vi "LV SCISDK Read Digitizer Data.vi"(8 "error in (no error)":errorcluster, 9 "handle":u64, 11 "Path":string) -> (0 "error out":errorcluster, 1 "handle out":u64, 2 "buffer out":T1, 3 "function return":i32)   [LabVIEW 2021, in "SciSDK_Labview.lvlib"]
doc: "SCISDKLABVIEW_DLL_API int LV_SCISDK_ReadDigitizer(char* Path, TD_DIGITIZER* buffer, void* handle);"
uses:
  SciSDK_Labview.lvlib
  SciSDK_VC++/x64/Debug/SciSDK_Labview.dll
panel:
  in  "buffer":T1={"magic"=0, "hits"=0, "timecode"=0, "counter"=0, "user"=0, "samples"=0, "valid_samples"=0, "channels"=0, "enabled_channels"=0, "analog"=[10, 100]}
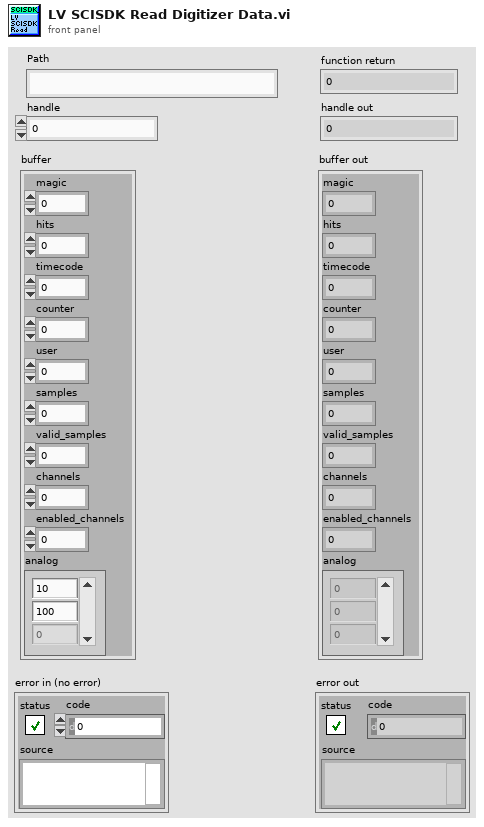
[diagram p1: front panel]
types:
  T1 = cluster{"magic":u32, "hits":u32, "timecode":u32, "counter":u32, "user":u32, "samples":u32, "valid_samples":u32, "channels":u32, "enabled_channels":u32, "analog":i32[]}
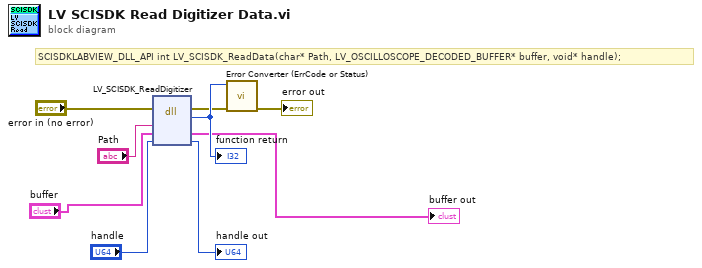
[diagram p0: block diagram]
diagram:
  # "SCISDKLABVIEW_DLL_API int LV_SCISDK_ReadData(char* Path, LV_OSCILLOSCOPE_DECODED_BUFFER* buffer, void* handle);"
  n1 = dll-call lib="C:/git/scisdk/SciSDK_VC++/x64/Debug/SciSDK_Labview.dll" fn="LV_SCISDK_ReadDigitizer"(error in="error in (no error)", "Path"="Path", "buffer"="buffer", "handle"="handle") -> (error out=w4:errorcluster, "return type"=w9:i32, "buffer"=→"buffer out":T1, "handle"=→"handle out":u64)  [unwired: 3 in, 1 out]
  "function return" <- w9
  n2 = call <userlib>:"Error Converter (ErrCode or Status).vi"("error in (no error)"=w4, "error code"=w9) -> ("error out"=→"error out":errorcluster)  [unwired: 9 in]
